vi "Parse Headers-Body.vi"(8 "error in":errorcluster, 11 "Header-Body Data in":T1) -> (0 "error out":errorcluster, 2 "HTTP Status":T2, 3 "Header-Body Data out":T1)   [LabVIEW 2020, in "InfluxDB v2 Client.lvlib"]
doc: "Parses headers and body into the components:\n1) Code\n2) Status (Headers)\n3) Status (Body)\n4) Desciption"
uses:
  InfluxDB v2 Client.lvlib
  HTTP Status.ctl
  Header-Body Data.ctl
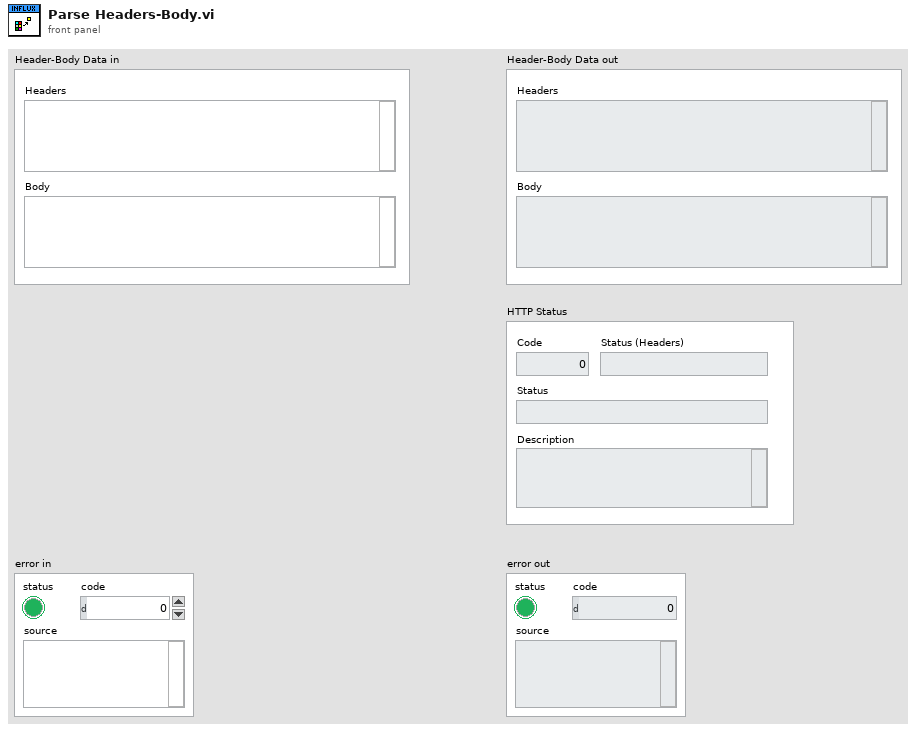
[diagram p1: front panel]
types:
  T1 = typedef "InfluxDB v2 Client.lvlib/Header-Body Data.ctl" = cluster{"Headers":string, "Body":string}
  T2 = typedef "InfluxDB v2 Client.lvlib/HTTP Status.ctl" = cluster{"Code":i32, "Status":string, "Description":string, "Status (Headers)":string}
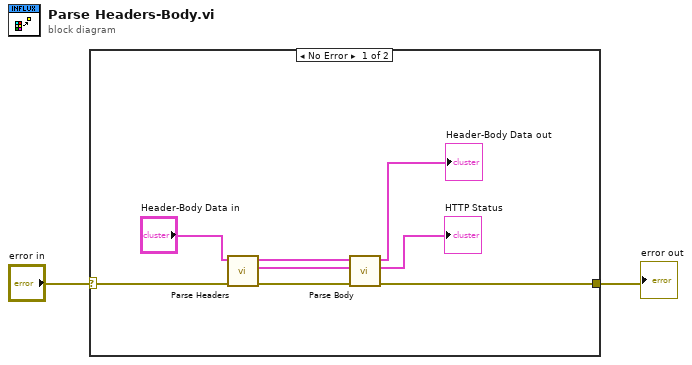
[diagram p0: block diagram]
diagram:
  n1 = case shown="No Error" "error in" {
    selector: "error in" -> [w10 w11]
    tunnel: [w5 w11] -> w1
    frame No Error {
      n2 = call "Parse Headers.vi"("error in"=w10, "Header-Body Data in"="Header-Body Data in") -> ("error out"=w9:errorcluster, "HTTP Status"=w6:T2, "Header-Body Data out"=w7:T1)  [unwired: 7 in]
      n3 = call "Parse Body.vi"("error in"=w9, "HTTP Status in"=w6, "Header-Body Data in"=w7) -> ("error out"=w5:errorcluster, "HTTP Status out"=→"HTTP Status":T2, "Header-Body Data out"=→"Header-Body Data out":T1)  [unwired: 6 in]
    }
    frame Error {
    }
  }
  "error out" <- w1
